vi "Clear.vi"(8 "error in (no error)":errorcluster, 11 "Collection in":refnum<class "CollectionByValue.lvclass">) -> (0 "error out":errorcluster, 3 "Collection out":refnum<class "CollectionByValue.lvclass">)   [LabVIEW 2021, in "Collection.lvlib" / "CollectionByValue.lvclass"]
uses:
  CollectionByValue.lvclass
  CollectionByValue.lvclass/CollectionByValue.ctl
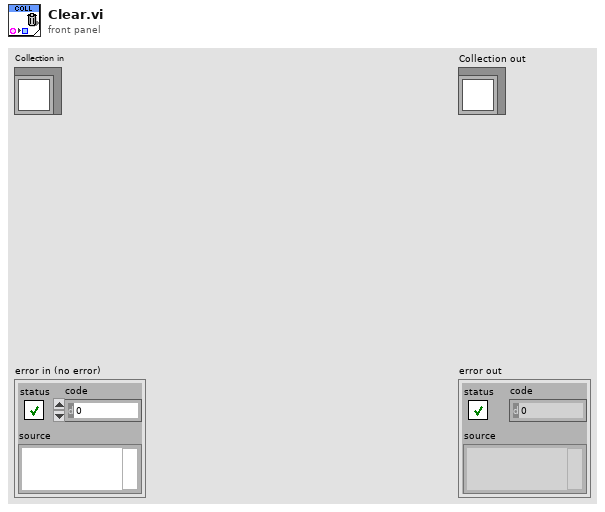
[diagram p1: front panel]
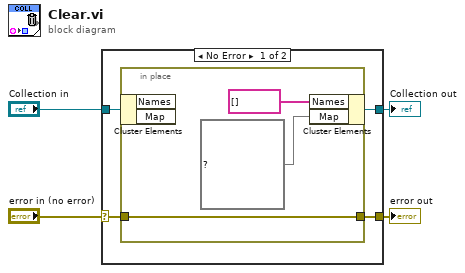
[diagram p0: block diagram]
diagram:
  n1 = case shown="No Error" "error in (no error)" {
    selector: "error in (no error)" -> [w6 w13]
    tunnel: [w5 w13] -> w3
    tunnel: [w7 w12] -> w1
    tunnel: "Collection in" -> [w8 w12]
    frame No Error {
      n2 = in-place {
        in-place-border: w6 -> [w10]
        in-place-border: [w10] -> w5
        n3 = in-place-cluster #1(w8) -> ()  [unwired: 2 out]
        n4 = in-place-cluster #1("Names"=string[] [], "Map"=map{string, refnum<class>} {}) -> (w7:refnum<class "CollectionByValue.lvclass">)
      }
    }
    frame Error {
    }
  }
  "error out" <- w3
  "Collection out" <- w1
